vi "tempcontrol.vi"() -> ()   [LabVIEW 2024]
uses:
  <vilib>/addons/control/pid/pid.llb/PID (DBL).vi
  <vilib>/addons/control/pid/NI_PID_pid.lvlib
panel:
  in  "stop":bool
  in  "PID gains":T1={"proportional gain (Kc)"=1.0, "integral time (Ti, min)"=0.01, "derivative time (Td, min)"=0.0} {"derivative time (Td, min)" format="%.3f"; "integral time (Ti, min)" format="%.3f"; "proportional gain (Kc)" format="%.3f"}
  in  "Running Average Temp":dbl
  in  "setpoint":dbl
  out "Heater status?":bool
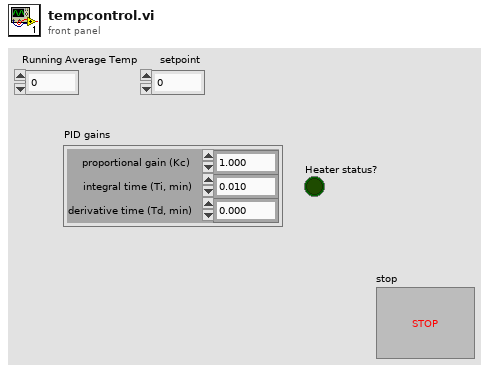
[diagram p1: front panel]
types:
  T1 = cluster{"proportional gain (Kc)":dbl, "integral time (Ti, min)":dbl, "derivative time (Td, min)":dbl}
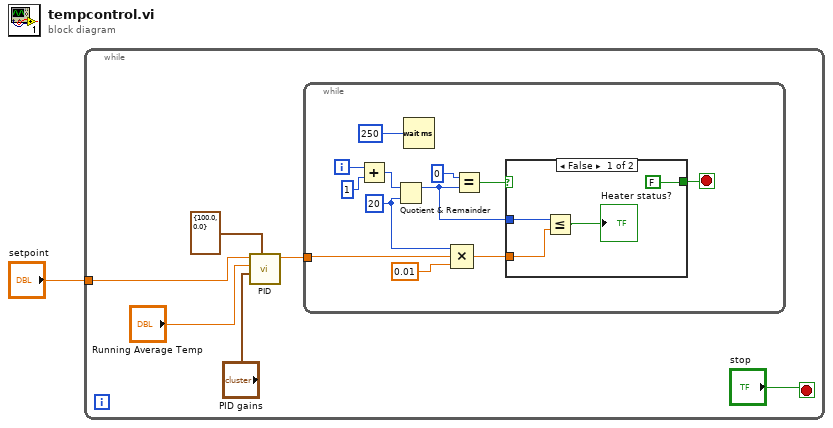
[diagram p0: block diagram]
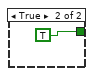
[diagram p2: hidden frame]
diagram:
  n1 = while {
    tunnel: "setpoint" -> [w2]
    stop <- "stop" stop-if-true
    n2 = call-poly <vilib>:"PID.vi"("output range"=cluster{"output high":dbl, "output low":dbl} {"output high"=100.0, "output low"=0.0}, "PID gains"="PID gains", "process variable"="Running Average Temp", "setpoint"=w2) -> ("output"=w6:dbl)  [unwired: 6 in, 1 out]
    n3 = while {
      tunnel: w6 -> [w17]
      i -> [w15]
      stop <- w10 stop-if-true
      w18 = 20 ("y")
      n4 = Add(x=w15, y=1) -> (x+y=w13:i32)
      n5 = Quotient & Remainder(x=w13, y=w18) -> (x-y*floor(x/y)=w9:i32)  [unwired: 1 out]
      n6 = Wait (ms)(milliseconds to wait=u32 250) -> ()  [unwired: 1 out]
      n7 = Compound Arithmetic op=MULTIPLY(w18, w17, 0.01 ("value")) -> (w8:dbl)
      n8 = Equal?(x=0, y=w9) -> (x = y?=w11:bool)
      n9 = case shown="False" w11 {
        tunnel: [FALSE TRUE] -> w10
        tunnel: w9 -> [w22 _]
        tunnel: w8 -> [w21 _]
        frame False {
          n10 = Less Or Equal?(x=w22, y=w21) -> (x <= y?=→"Heater status?":bool)
        }
        frame True {
        }
      }
    }
  }
